vi "Simulated Active DTCs.vi"() -> (3 "payload":u8[](array[numeric]))   [LabVIEW 2013, in "J1939.lvlib"]
uses:
  J1939.lvlib
  API Types/Convert DTCs Cluster.ctl
  <vilib>/xnet/xnet.llb/XNET Frame CAN.ctl
  <vilib>/xnet/xnet.llb/XNET Frame Type CAN.ctl
panel:
  out "Converted Value":T1={"Lamps"={"Malfunction Indicator"=0, "Red Stop"=0, "Amber Warning"=2, "Protect Lamp"=1}, "DTCs"=[{"SPN"=4625, "FMI"=19, "Occurrance"=20}, {"SPN"=5653, "FMI"=23, "Occurrance"=24}, {"SPN"=73753, "FMI"=1, "Occurrance"=34}], "Active?"=FALSE, "Address"=0, "timestamp"=timestamp(0 s since 1904-01-01)}
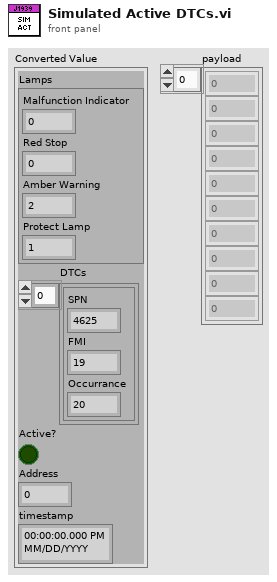
[diagram p1: front panel]
types:
  T1 = typedef "J1939.lvlib/Convert DTCs Cluster.ctl" = cluster{"Lamps":cluster{"Malfunction Indicator":u8, "Red Stop":u8, "Amber Warning":u8, "Protect Lamp":u8}, "DTCs":cluster{"SPN":u32, "FMI":u8, "Occurrance":u8}[], "Active?":bool, "Address":u8, "timestamp":timestamp}
  T2 = typedef "XNET Frame CAN.ctl" = cluster{"timestamp":timestamp, "payload":u8[], "identifier":u32, "type":T3, "extended?":bool, "echo?":bool}
  T3 = typedef "XNET Frame Type CAN.ctl" = u8
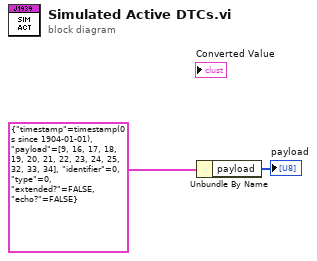
[diagram p0: block diagram]
diagram:
  n1 = Unbundle By Name(T2 {"timestamp"=timestamp(0 s since 1904-01-01), "payload"=[9, 16, 17, 18, 19, 20, 21, 22, 23, 24, 25, 32, 33, 34], "identifier"=0, "type"=0, "extended?"=FALSE, "echo?"=FALSE} ("Value")) -> ("payload"=→"payload":u8[])
